vi "Create ProcessData Q.vi"(8 "error in (no error)":errorcluster, 10 "Processing loop variables":T1 {"CurrInverter"."last updated" format="%<%H:%M\n%d/%m/%Y>T"; "CurrInverter"."set flag" items=["False", "True"]}, 11 "QName":string) -> (0 "error out":errorcluster, 3 "ProcDataQRef":refnum<queue>)   [LabVIEW 2019]
doc: "Developed by Kevin Thompson\nThompson Engineering, LLC\nkevin@thompsonengineering.net"
uses:
  GBL DataQ Ref.vi
  Subsystems/Main/support/Data Algorithms/subvis/DataTypes/averaging variables.ctl
  Subsystems/Main/Main.lvclass
  Subsystems/Main/support/Data Algorithms/subvis/DataTypes/ESR alarm variables.ctl
  Subsystems/Main/support/Data Algorithms/subvis/DataTypes/Processing loop variables--cluster.ctl
  DataTypes/inverter gain range--cluster.ctl
  DataTypes/inverter offset range--cluster.ctl
  DataTypes/inverter info v2--cluster.ctl
  DataTypes/Inverter database record v2--cluster.ctl
panel:
  out "data reference":u32
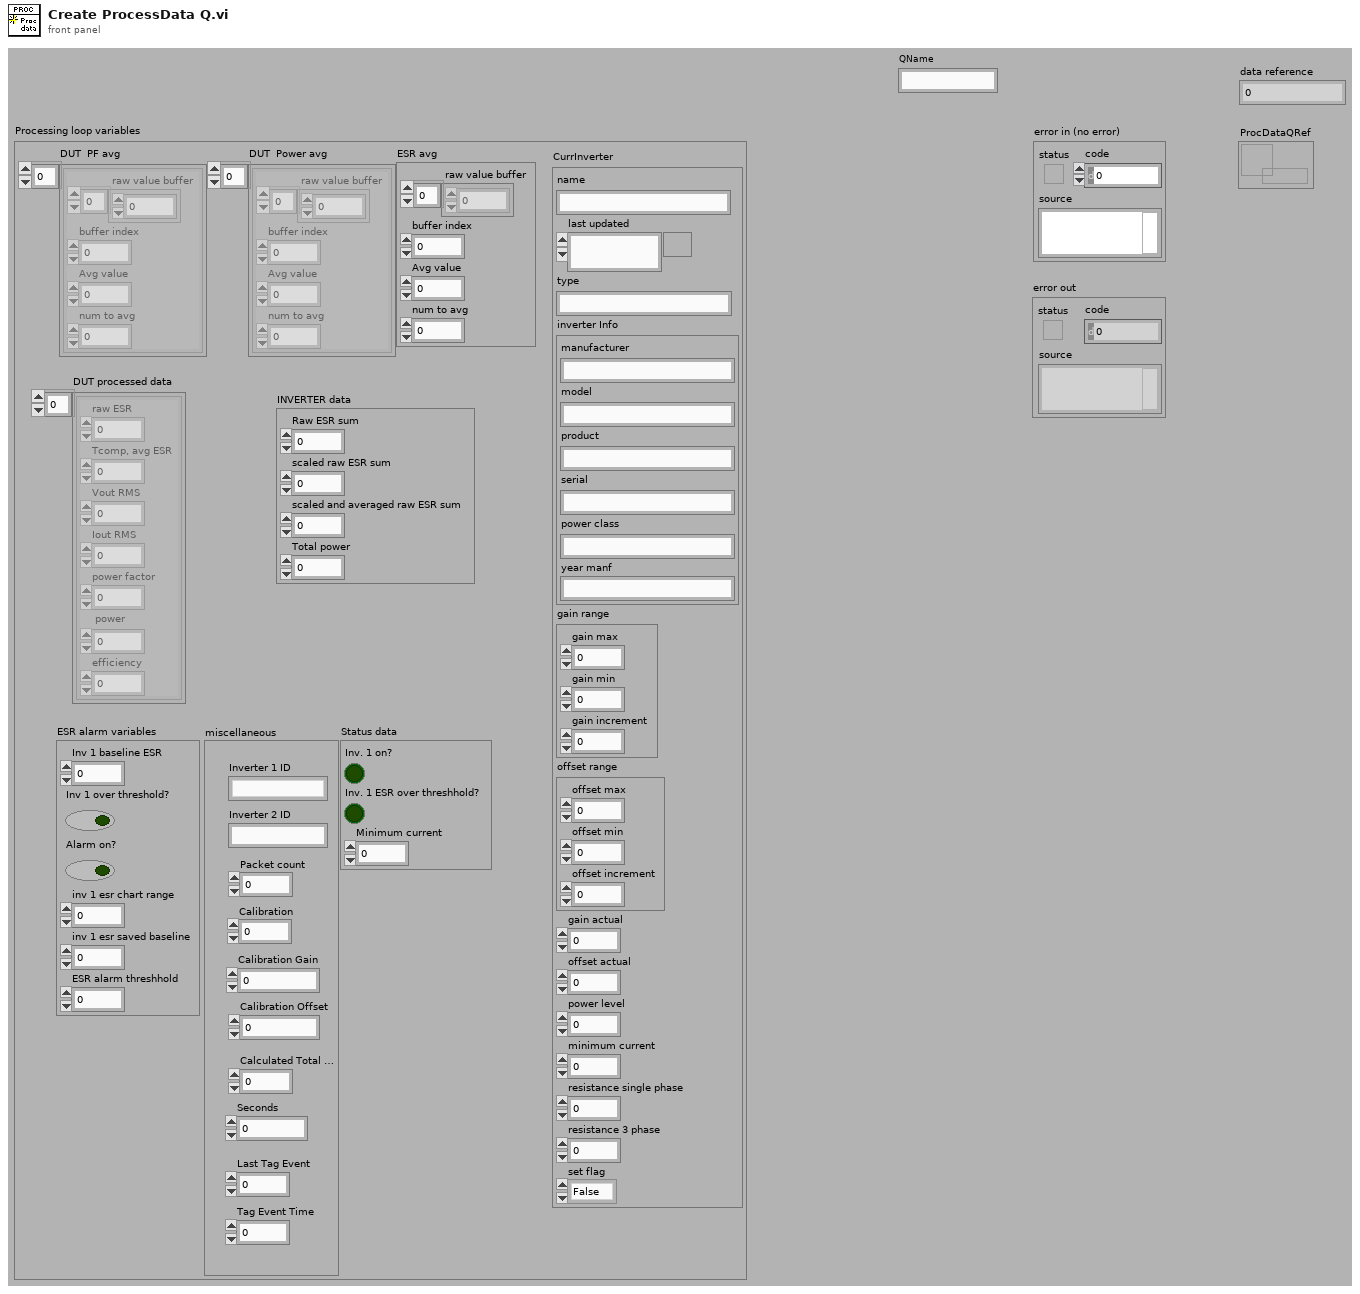
[diagram p1: front panel]
types:
  T1 = typedef "Main.lvclass/Processing loop variables--cluster.ctl" = cluster{"ESR avg":T2, "DUT  PF avg":T2[], "DUT  Power avg ":T2[], "INVERTER data":cluster{"Raw ESR sum":dbl, "scaled raw ESR sum":dbl, "scaled and averaged raw ESR sum":dbl, "Total power":dbl}, "DUT processed data":cluster{"raw ESR":dbl, "Tcomp, avg ESR":dbl, "Vout RMS":dbl, "Iout RMS":dbl, "power factor":dbl, "power":dbl, "efficiency":dbl}[], "ESR alarm variables":T3, "Status data":cluster{"Inv. 1 on?":bool, "Inv. 1 ESR over threshhold?":bool, "Minimum current":dbl}, "CurrInverter":T4, "miscellaneous":cluster{"Inverter 1 ID":string, "Inverter 2 ID":string, "Packet count":u32, "Calibration":dbl, "Calibration Gain":dbl, "Calibration Offset":dbl, "Calculated Total Power":dbl, "Seconds":dbl, "Last Tag Event":dbl, "Tag Event Time":dbl}}
  T2 = typedef "Main.lvclass/averaging variables.ctl" = cluster{"raw value buffer":dbl[], "buffer index":i32, "Avg value":dbl, "num to avg":i32}
  T3 = typedef "Main.lvclass/ESR alarm variables.ctl" = cluster{"Inv 1 baseline ESR":dbl, "Inv 1 over threshold?":bool, "Alarm on?":bool, "inv 1 esr chart range":dbl, "inv 1 esr saved baseline":dbl, "ESR alarm threshhold":dbl}
  T4 = typedef "Inverter database record v2--cluster.ctl" = cluster{"name":string, "last updated":timestamp, "type":string, "inverter Info":T5, "gain range":T6, "offset range":T7, "gain actual":dbl, "offset actual":dbl, "power level":dbl, "minimum current":dbl, "resistance single phase":dbl, "resistance 3 phase":dbl, "set flag":u16}
  T5 = typedef "inverter info v2--cluster.ctl" = cluster{"manufacturer":string, "model":string, "product":string, "serial":string, "power class":string, "year manf":string}
  T6 = typedef "inverter gain range--cluster.ctl" = cluster{"gain max":dbl, "gain min":dbl, "gain increment":dbl}
  T7 = typedef "inverter offset range--cluster.ctl" = cluster{"offset max":dbl, "offset min":dbl, "offset increment":dbl}
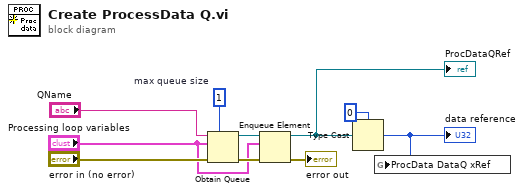
[diagram p0: block diagram]
diagram:
  w9 = 1  # max queue size
  n1 = Obtain Queue(max queue size (-1, unlimited)=w9, name (unnamed)="QName", element data type="Processing loop variables", error in (no error)="error in (no error)") -> (queue out=w6:refnum<queue>, error out=w7:errorcluster)  [unwired: 1 in, 1 out]
  n2 = Enqueue Element(queue=w6, element="Processing loop variables", error in (no error)=w7) -> (queue out=w3:refnum<queue>, error out=→"error out":errorcluster)  [unwired: 1 in, 1 out]
  "ProcDataQRef" <- w3
  n3 = Type Cast(type=u32 0, x=w3) -> (*(type *) &x=w1:u32)
  "data reference" <- w1
  n4 = global write "GBL DataQ Ref.vi" "ProcData DataQ xRef"(w1) -> ()
